vi "Complement.vi"() -> ()   [LabVIEW 2014, in "ALPHA5 RS485.lvlib"]
uses:
  ALPHA5 RS485.lvlib
panel:
  out "32bit integer":i32
  out "unsigned 32bit integer":u32 format="%.0x"
  in  "Parse Complement":u32
  in  "Cal Complement":i32 format="%.0x"
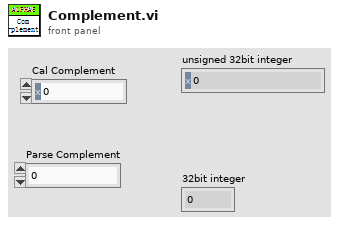
[diagram p1: front panel]
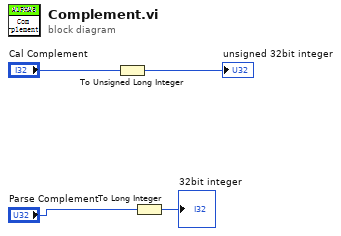
[diagram p0: block diagram]
diagram:
  n1 = To Unsigned Long Integer(number="Cal Complement") -> (unsigned 32bit integer=→"unsigned 32bit integer":u32)
  n2 = To Long Integer(number="Parse Complement") -> (32bit integer=→"32bit integer":i32)
